vi "Unlock SPAN Registers.vi"() -> (3 "Array":string[](array[string]))   [LabVIEW 2020, in "Linearisierung v2.lvlib" / "SpanEinstellungen.lvlib"]
uses:
  SpanEinstellungen.lvlib
  Aktion FGV SpanEinstellungen.ctl
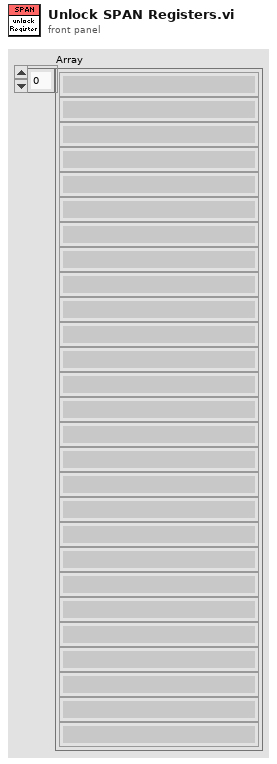
[diagram p1: front panel]
types:
  T1 = enum8{"Enabled", "Disabled", "Disabled and Grayed Out"}
  T2 = typedef "Linearisierung v2.lvlib/SpanEinstellungen.lvlib/Aktion FGV SpanEinstellungen.ctl" = enum16{"lesen", "schreiben", "laden", "speichern", "RegisterRef", "automatisch", "init", "PDF Params", "Punkte umkehren"}
  T3 = cluster{"HauptRegister in":refnum<vi>, "SpanRegister in":refnum<vi>}
  T4 = typedef "System Einstellungen V2.lvlib/Konfig Gasflasche.ctl" = bool
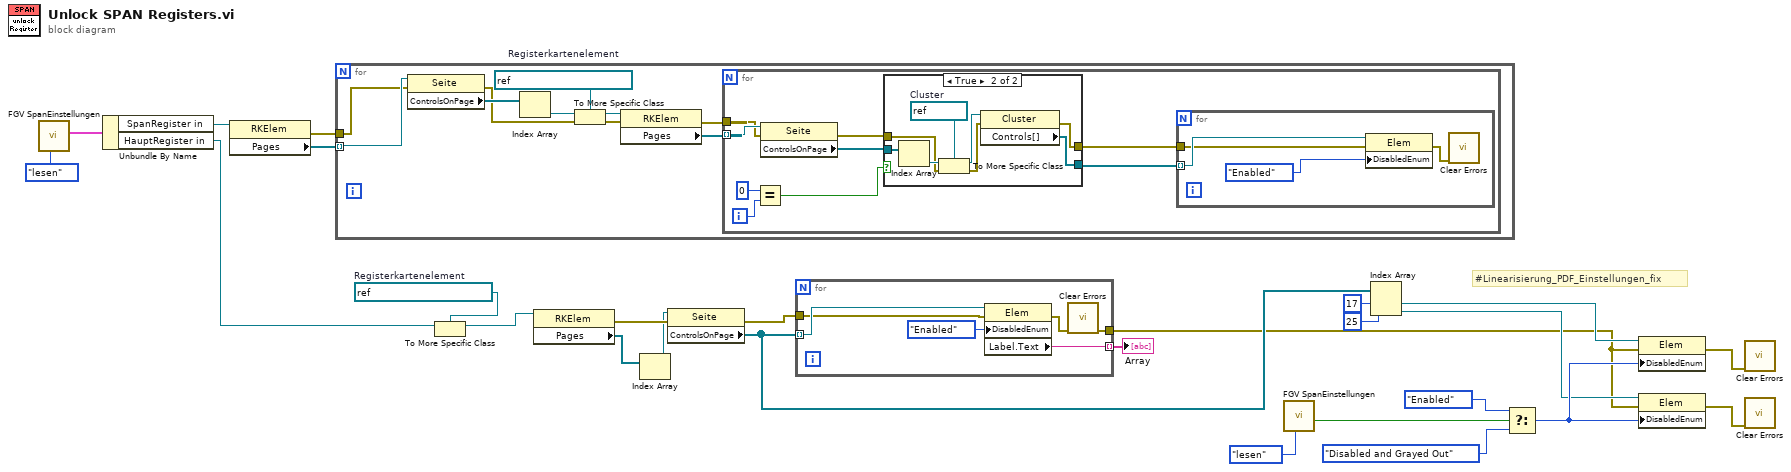
[diagram p0: block diagram]
diagram:
  w23 = refnum<vi> refnum  # Registerkartenelement
  # "#Linearisierung_PDF_Einstellungen_fix"
  n1 = call "FGV SpanEinstellungen.vi"("Aktion"=Aktion_FGV_SpanEinstellungen."lesen") -> ("RegisterRefs out"=w17:T3)  [unwired: 6 in, 4 out]
  n2 = Unbundle By Name(w17) -> ("SpanRegister in"=w16:refnum<vi>, "HauptRegister in"=w15:refnum<vi>)
  n3 = property class="RKElem"(reference=w16) -> (error out=w25:errorcluster, "Pages"=w24:refnum<vi>[])  [unwired: 1 in, 1 out]
  n4 = for {
    tunnel: w24 -> [w36] mode=indexing
    tunnel: w25 -> [w29]
    w33 = refnum<vi> refnum  # Registerkartenelement
    n5 = property class="Seite"(reference=w36, error in=w29) -> (error out=w30:errorcluster, "ControlsOnPage"=w35:refnum<vi>[])  [unwired: 1 out]
    n6 = Index Array(array=w35) -> (element=w34:refnum<vi>)  [unwired: 1 in]
    n7 = To More Specific Class(target class=w33, reference=w34, error in=w30) -> (specific class reference=w32:refnum<vi>, error out=w31:errorcluster)
    n8 = property class="RKElem"(reference=w32, error in=w31) -> (error out=w27:errorcluster, "Pages"=w28:refnum<vi>[])  [unwired: 1 out]
    n9 = for {
      tunnel: w28 -> [w45] mode=indexing
      tunnel: w27 -> [w44]
      i -> [w38]
      n10 = Equal?(x=0, y=w38) -> (x = y?=w37:bool)
      n11 = property class="Seite"(reference=w45, error in=w44) -> (error out=w43:errorcluster, "ControlsOnPage"=w41:refnum<vi>[])  [unwired: 1 out]
      n12 = case shown="True" w37 {
        tunnel: w43 -> [w46 w52]
        tunnel: [w46 w55] -> w42
        tunnel: w41 -> [w47 w54]
        tunnel: [w47 w48] -> w40
        frame False {
        }
        frame True {
          w50 = refnum<vi> refnum  # Cluster
          n13 = Index Array(array=w54) -> (element=w53:refnum<vi>)  [unwired: 1 in]
          n14 = To More Specific Class(target class=w50, reference=w53, error in=w52) -> (specific class reference=w49:refnum<vi>, error out=w51:errorcluster)
          n15 = property class="Cluster"(reference=w49, error in=w51) -> (error out=w55:errorcluster, "Controls[]"=w48:refnum<vi>[])  [unwired: 1 out]
        }
      }
      n16 = for {
        tunnel: w40 -> [w59] mode=indexing
        tunnel: w42 -> [w58]
        n17 = property class="Elem"(reference=w59, error in=w58, "DisabledEnum"=T1."Enabled" ("Deaktiviert")) -> (error out=w57:errorcluster)  [unwired: 1 out]
        n18 = call <vilib>:"Clear Errors.vi"("error in (no error)"=w57) -> ()  [unwired: 5 in, 2 out]
      }
    }
  }
  n19 = To More Specific Class(target class=w23, reference=w15) -> (specific class reference=w22:refnum<vi>)  [unwired: 1 in, 1 out]
  n20 = property class="RKElem"(reference=w22) -> (error out=w21:errorcluster, "Pages"=w20:refnum<vi>[])  [unwired: 1 in, 1 out]
  n21 = Index Array(array=w20) -> (element=w19:refnum<vi>)  [unwired: 1 in]
  n22 = property class="Seite"(reference=w19, error in=w21) -> (error out=w18:errorcluster, "ControlsOnPage"=w6:refnum<vi>[])  [unwired: 1 out]
  n23 = for {
    tunnel: w6 -> [w65] mode=indexing
    tunnel: w18 -> [w63]
    tunnel: [w61] -> w14 mode=indexing
    tunnel: [w60] -> w1
    n24 = property class="Elem"(reference=w65, error in=w63, "DisabledEnum"=T1."Enabled" ("Deaktiviert")) -> (error out=w62:errorcluster, "Label.Text"=w61:string)  [unwired: 1 out]
    n25 = call <vilib>:"Clear Errors.vi"("error in (no error)"=w62) -> ("error out"=w60:errorcluster)  [unwired: 5 in, 1 out]
  }
  "Array" <- w14
  n26 = call "FGV SpanEinstellungen.vi"("Aktion"=Aktion_FGV_SpanEinstellungen."lesen") -> ("automatisch out"=w12:T4)  [unwired: 6 in, 4 out]
  n27 = Index Array(array=w6, index #1=17 ("Index"), index #2=25 ("Index")) -> (element #1=w5:refnum<vi>, element #2=w4:refnum<vi>)
  n28 = Select(t=T1."Enabled", s=w12, f=T1."Disabled and Grayed Out" ("Deaktiviert")) -> (s? t:f=w7:T1)
  n29 = property class="Elem"(reference=w5, error in=w1, "DisabledEnum"=w7) -> (error out=w8:errorcluster)  [unwired: 1 out]
  n30 = property class="Elem"(reference=w4, error in=w1, "DisabledEnum"=w7) -> (error out=w9:errorcluster)  [unwired: 1 out]
  n31 = call <vilib>:"Clear Errors.vi"("error in (no error)"=w8) -> ()  [unwired: 5 in, 2 out]
  n32 = call <vilib>:"Clear Errors.vi"("error in (no error)"=w9) -> ()  [unwired: 5 in, 2 out]
